vi "Select Folder , File Name.vi"(1 "OK Button":bool, 2 "File Name":string) -> (0 "concatenated string":string)   [LabVIEW 2014]
panel:
  out "x = y?":bool
  out "ButtonPressed":i32(ring) items=["None", "OK", "Cancel", "Abort", "Retry", "Ignore", "Yes", "No"]
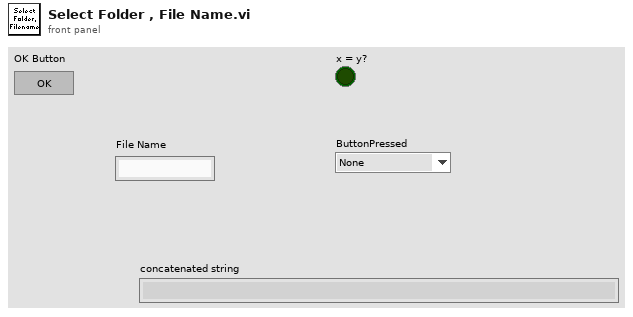
[diagram p1: front panel]
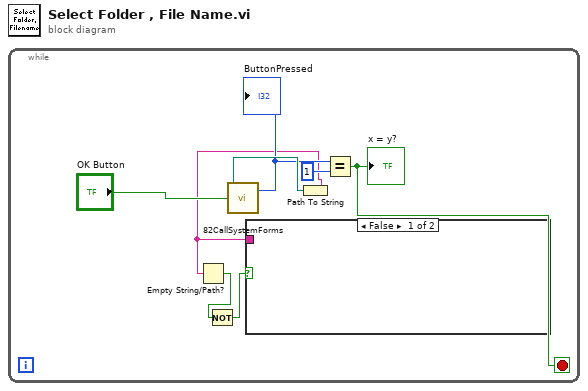
[diagram p0: block diagram]
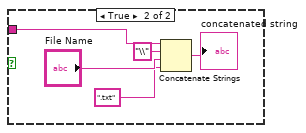
[diagram p2: hidden frame]
diagram:
  n1 = while {
    stop <- w7 stop-if-true
    n2 = call "82CallSystemForms.vi"("OK Button"="OK Button") -> ("ButtonPressed"=w5:i32, "Path"=w6:path)  [unwired: 1 in, 1 out]
    "ButtonPressed" <- w5
    n3 = Path To String(path=w6) -> (string=w1:string)
    n4 = Empty String/Path?(string/path=w1) -> (empty?=w3:bool)
    n5 = Not(x=w3) -> (.not. x?=w2:bool)
    n6 = case shown="False" w2 {
      tunnel: w1 -> [_ w9]
      frame False {
      }
      frame True {
        n7 = Concatenate Strings(w9, "\\" ("string"), "File Name", ".txt") -> (→"concatenated string":string)
      }
    }
    n8 = Equal?(x=w5, y=1) -> (x = y?=w7:bool)
    "x = y?" <- w7
  }
